vi "read qualified channel list.vi"(11 "module configuration in":refnum<class "TBM module configuration.lvclass">) -> (2 "qualified channels":refnum<class "TBM channel.lvclass">[](array[class]), 3 "module configuration out":refnum<class "TBM module configuration.lvclass">)   [LabVIEW 2013, in "TBM module configuration.lvclass"]
doc: "This function returns all configured channels in the system, qualified by the instance name. Children may override this function to provide additional path information. For example, while the default implementation might return channels of the form \"scan engine module/ai0\", that module may want to instead return \"scan engine module/mod1/ai0\"."
uses:
  TBM module configuration.lvclass
  channel/TBM channel.lvclass
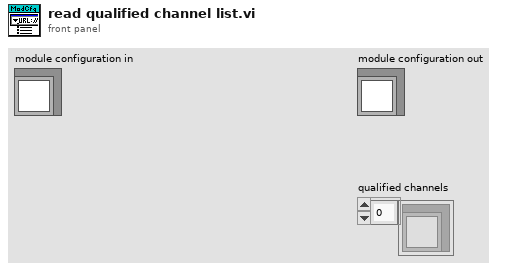
[diagram p1: front panel]
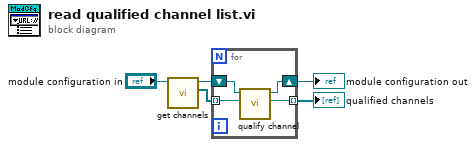
[diagram p0: block diagram]
diagram:
  n1 = call-dynamic "get channels.vi"("module configuration in"="module configuration in") -> ("channels"=w4:refnum<class "TBM channel.lvclass">[], "module configuration out"=w3:refnum<class "TBM module configuration.lvclass">)  [unwired: 9 in]
  n2 = for {
    tunnel: w4 -> [w6] mode=indexing
    shift-right: [w8] -> w2
    shift-left: w3 -> [w9]
    tunnel: [w7] -> w1 mode=indexing
    n3 = call "qualify channel.vi"("unqualified channel"=w6, "module configuration in"=w9) -> ("qualified channel"=w7:refnum<class "TBM channel.lvclass">, "module configuration out"=w8:refnum<class "TBM module configuration.lvclass">)  [unwired: 8 in]
  }
  "module configuration out" <- w2
  "qualified channels" <- w1
